vi "Open_tdms.vi"(11 "Folder path":path) -> (0 "error out":errorcluster, 3 "tdms refnum out":refnum<k34>, 4 "New log file path":path)   [LabVIEW 2017, in "labview-standard-library.lvlib" / "data-logging.lvlib"]
uses:
  data-logging.lvlib
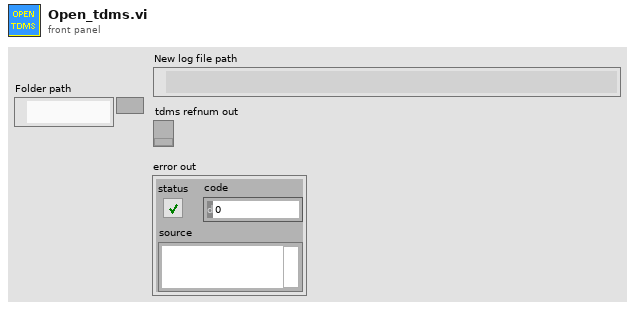
[diagram p1: front panel]
types:
  T1 = enum16{"open", "open or create", "create or replace", "create", "open (read-only)"}
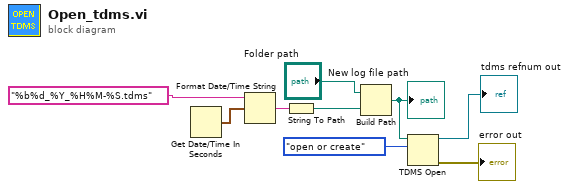
[diagram p0: block diagram]
diagram:
  n1 = Get Date/Time In Seconds() -> (seconds since 1Jan1904=w9:timestamp)
  n2 = Format Date/Time String(time format string (%c)="%b%d_%Y_%H%M-%S.tdms", seconds (now)=w9) -> (date/time string=w6:string)  [unwired: 1 in]
  n3 = String To Path(string=w6) -> (path=w7:path)
  n4 = Build Path(base path="Folder path", name or relative path=w7) -> (appended path=w4:path)
  "New log file path" <- w4
  n5 = TDMS Open(10:T1."open or create" ("operation (0:open)"), 11:w4) -> (0:→"error out":errorcluster, 3:→"tdms refnum out":refnum<k34>)  [unwired: 5 in]
